vi "Check for Mapping Conflicts.vi"(8 "error in (no error)":errorcluster, 10 "Type":T3, 11 "Coiil Group Ref in in":T1 format="%.0x") -> (0 "error out":errorcluster, 1 "Conflicts?":bool, 2 "Array":T2(array[cluster]), 3 "Coiil Group Ref out":T1 format="%.0x")   [LabVIEW 2021, in "Modbus Master System Explorer.lvlib"]
uses:
  Modbus Master System Explorer.lvlib
  SubVIs/Modbus Type.ctl
  <vilib>/NI VeriStand/Custom Device API/Custom Device Item Ref.ctl
  <vilib>/NI VeriStand/Custom Device API/Custom Device API.lvlib
  Shared/Modbus Master Shared.lvlib
panel:
  out "Conflicting":cluster{"y":i32, "y 2":i32, "Mapping":u16}[](array[cluster])
  out "Starting Address":u16[](array[numeric])
  out "Unit ID":u8[](array[numeric])
  # "Debugging Only"
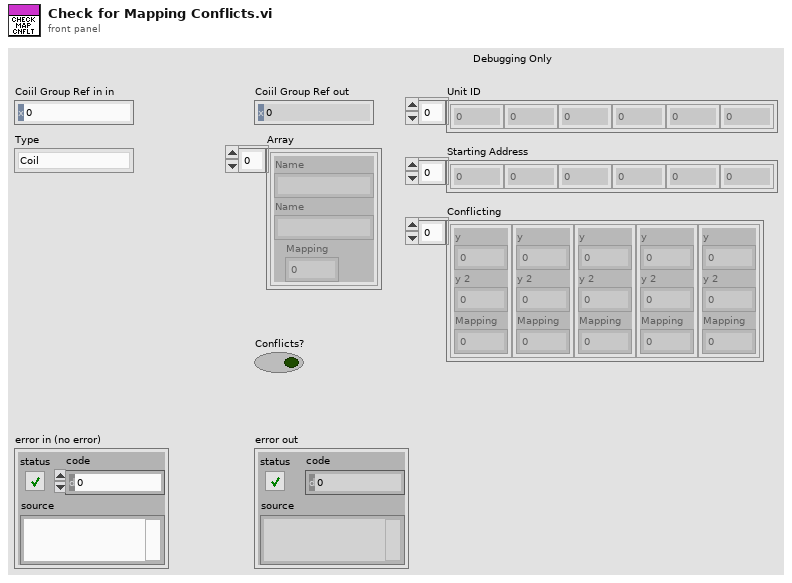
[diagram p1: front panel]
types:
  T1 = typedef "Custom Device API.lvlib/Custom Device Item Ref.ctl" = u64
  T2 = cluster{"Name":string, "Name":string, "Mapping":u16}[]
  T3 = typedef "Modbus Master Shared.lvlib/Modbus Type.ctl" = enum16{"Coil", "Discrete Input", "Holding Register", "Input Register"}
  T4 = typedef "Modbus Master Shared.lvlib/Mapping.ctl" = cluster{"DataType":T5, "Unit ID":u8, "Starting Address":u16, "Sub-Index (Bool)":u16, "VS Reference":T1}
  T5 = typedef "Modbus Master Shared.lvlib/DataType.ctl" = enum16{"Double", "Single", "I64", "I32", "I16", "I8", "U64", "U32", "U16", "U8", "Boolean"}
  T6 = typedef "Custom Device API.lvlib/Custom Device Item Info.ctl" = cluster{"Name":string, "Is Channel":bool, "GUID":string, "Is Waveform":bool}
  T7 = cluster{"Name":string, "Name":string, "Mapping":u16}
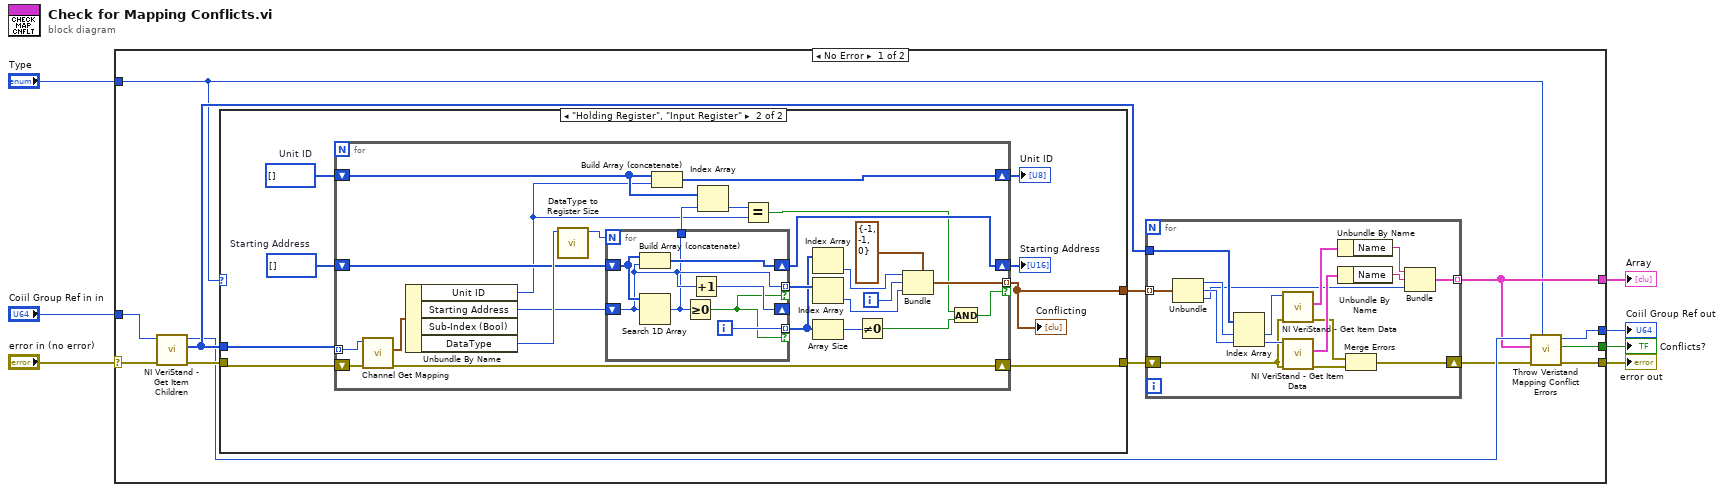
[diagram p0: block diagram]
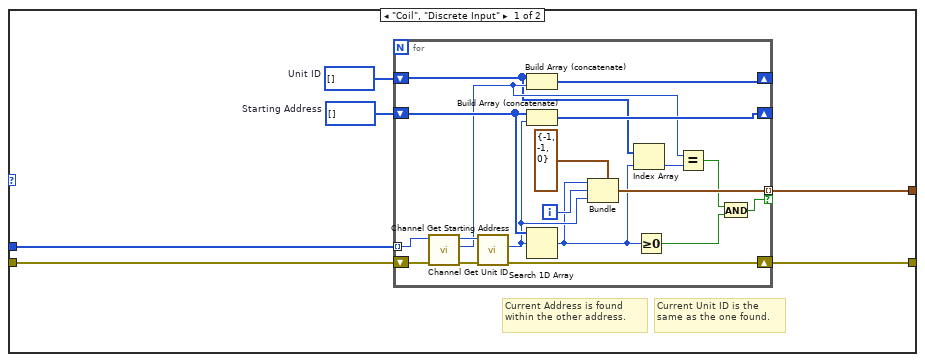
[diagram p2: hidden frame]
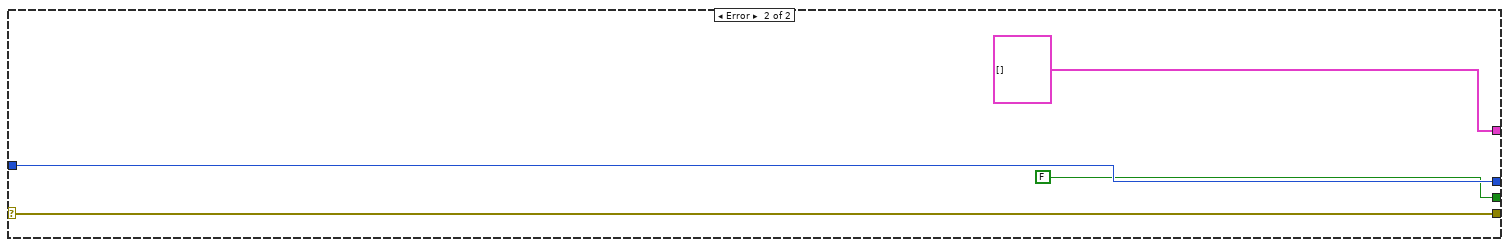
[diagram p3: hidden frame]
diagram:
  n1 = case shown="No Error" "error in (no error)" {
    selector: "error in (no error)" -> [w17 w104]
    tunnel: "Coiil Group Ref in in" -> [w18 w105]
    tunnel: [w14 w105] -> w3
    tunnel: [w12 T2 []] -> w4
    tunnel: [w10 w104] -> w5
    tunnel: [w9 FALSE ("Conflicts?")] -> w6
    tunnel: "Type" -> [w8 _]
    frame No Error {
      n2 = call <vilib>:"NI VeriStand - Get Item Children.vi"("error in (no error)"=w17, "Item Ref in"=w18) -> ("error out"=w16:errorcluster, "Child Refs"=w20:T1[], "Item Ref out"=w13:T1)  [unwired: 6 in, 1 out]
      n3 = case shown="\"Holding Register\", \"Input Register\"" w8 {
        tunnel: w20 -> [w26 w49]
        tunnel: [w25 w50] -> w19
        tunnel: w16 -> [w23 w48]
        tunnel: [w22 w51] -> w15
        frame "Coil", "Discrete Input" {
          w21 = u8[] []  # Unit ID
          w24 = u16[] []  # Starting Address
          # "Current Unit ID is the same as the one found."
          # "Current Address is found within the other address."
          n4 = for {
            tunnel: w26 -> [w35] mode=indexing
            shift-right: [w45] -> _
            shift-left: w24 -> [w44]
            tunnel: [w42] -> w25 mode=indexing if=w33
            shift-right: [w39] -> w22
            shift-left: w23 -> [w38]
            shift-right: [w32] -> _
            shift-left: w21 -> [w28]
            i -> [w41]
            n5 = call "Channel Get Unit ID.vi"("error in (no error)"=w38, "Item Ref in"=w35) -> ("error out"=w37:errorcluster, "Value"=w29:u8, "Item Ref out"=w36:T1)  [unwired: 7 in]
            n6 = call "Channel Get Starting Address.vi"("error in (no error)"=w37, "Item Ref in"=w36) -> ("error out"=w39:errorcluster, "Value"=w40:u16)  [unwired: 7 in, 1 out]
            n7 = Build Array (concatenate)(w28, w29) -> (w32:u8[])
            n8 = Build Array (concatenate)(w44, w40) -> (w45:u16[])
            n9 = Search 1D Array(1D array=w44, element=w40) -> (index of element=w31:i32)  [unwired: 1 in]
            n10 = Bundle(cluster=cluster{"y":i32, "y 2":i32, "Mapping":u16} {"y"=-1, "y 2"=-1, "Mapping"=0} ("Conflicting Indices"), "y"=w31, "y 2"=w41, "Mapping"=w40) -> (w42:cluster{"y":i32, "y 2":i32, "Mapping":u16})
            n11 = Index Array(array=w28, index=w31) -> (element=w30:u8)
            n12 = Greater Or Equal To 0?(x=w31) -> (x >= 0?=w34:bool)
            n13 = Equal?(x=w29, y=w30) -> (x = y?=w27:bool)
            n14 = And(x=w27, y=w34) -> (x .and. y?=w33:bool)
          }
        }
        frame "Holding Register", "Input Register" {
          w52 = u8[] []  # Unit ID
          w53 = u16[] []  # Starting Address
          n15 = for {
            shift-right: [w71] -> w46
            shift-left: w53 -> [w72]
            tunnel: [w77] -> w50 mode=indexing if=w54
            tunnel: w49 -> [w64] mode=indexing
            shift-right: [w62] -> w51
            shift-left: w48 -> [w63]
            shift-right: [w61] -> w47
            shift-left: w52 -> [w59]
            i -> [w76]
            n16 = call "Channel Get Mapping.vi"("error in (no error)"=w63, "Item Ref in"=w64) -> ("error out"=w62:errorcluster, "Mapping"=w65:T4)  [unwired: 7 in, 1 out]
            n17 = Unbundle By Name(w65) -> ("Unit ID"=w57:u8, "Starting Address"=w73:u16, "DataType"=w75:T5)  [unwired: 1 out]
            n18 = call "DataType to Register Size.vi"("DataType"=w75) -> ("Registers"=w74:i32)  [unwired: 9 in, 1 out]
            n19 = for {
              N: w74 -> [_]
              shift-right: [w83] -> w71
              shift-left: w72 -> [w85]
              shift-right: [w84] -> _
              shift-left: w73 -> [w82]
              tunnel: [w81] -> w67 mode=indexing if=w80
              tunnel: [w82] -> w69 mode=indexing if=w80
              tunnel: [w79] -> w60
              i -> [w81]
              n20 = Build Array (concatenate)(w85, w82) -> (w83:u16[])
              n21 = Search 1D Array(1D array=w85, element=w82) -> (index of element=w79:i32)  [unwired: 1 in]
              n22 = Greater Or Equal To 0?(x=w79) -> (x >= 0?=w80:bool)
              n23 = Increment(x=w82) -> (x+1=w84:u16)
            }
            n24 = Build Array (concatenate)(w59, w57) -> (w61:u8[])
            n25 = Index Array(array=w59, index=w60) -> (element=w58:u8)
            n26 = Equal?(x=w58, y=w57) -> (x = y?=w56:bool)
            n27 = Index Array(array=w67) -> (element=w66:i32)  [unwired: 1 in]
            n28 = Index Array(array=w69) -> (element=w68:u16)  [unwired: 1 in]
            n29 = Array Size(array=w67) -> (size(s)=w70:i32)
            n30 = Not Equal To 0?(x=w70) -> (x != 0?=w55:bool)
            n31 = Bundle(cluster=cluster{"y":i32, "y 2":i32, "Mapping":u16} {"y"=-1, "y 2"=-1, "Mapping"=0} ("Conflicting Indices"), "y"=w66, "y 2"=w76, "Mapping"=w68) -> (w77:cluster{"y":i32, "y 2":i32, "Mapping":u16})
            n32 = And(x=w56, y=w55) -> (x .and. y?=w54:bool)
          }
          "Unit ID" <- w47
          "Starting Address" <- w46
          "Conflicting" <- w50
        }
      }
      n33 = for {
        tunnel: w19 -> [w101] mode=indexing
        tunnel: w20 -> [w100]
        tunnel: [w91] -> w12 mode=indexing
        shift-right: [w86] -> w11
        shift-left: w15 -> [w89]
        n34 = Unbundle(w101) -> ("y"=w99:i32, "y 2"=w98:i32, "Mapping"=w90:u16)
        n35 = Index Array(array=w100, index #1=w99, index #2=w98) -> (element #1=w97:T1, element #2=w96:T1)
        n36 = call <vilib>:"NI VeriStand - Get Item Data.vi"("error in (no error)"=w89, "Item Ref in"=w97) -> ("error out"=w88:errorcluster, "Item Info"=w95:T6)  [unwired: 8 out]
        n37 = call <vilib>:"NI VeriStand - Get Item Data.vi"("error in (no error)"=w89, "Item Ref in"=w96) -> ("error out"=w87:errorcluster, "Item Info"=w94:T6)  [unwired: 8 out]
        n38 = Unbundle By Name(w95) -> ("Name"=w93:string)
        n39 = Unbundle By Name(w94) -> ("Name"=w92:string)
        n40 = Merge Errors(w88, w87) -> (w86:errorcluster)
        n41 = Bundle("Name"=w93, "Name"=w92, "Mapping"=w90) -> (w91:T7)  [unwired: 1 in]
      }
      n42 = call "Throw Veristand Mapping Conflict Errors.vi"("Type"=w8, "error in (no error)"=w11, "Conflicts In"=w12, "Item Ref in"=w13) -> ("error out"=w10:errorcluster, "Conflicts?"=w9:bool, "Node Ref out"=w14:T1)  [unwired: 5 in]
    }
    frame Error {
    }
  }
  "Conflicts?" <- w6
  "error out" <- w5
  "Array" <- w4
  "Coiil Group Ref out" <- w3
